vi "Actuator.vi"(10 "Actuator":bool, 11 "lines":tag) -> ()   [LabVIEW 2016]
uses:
  <vilib>/DAQmx/write.llb/DAQmx Write (Digital Bool 1Line 1Point).vi
  <vilib>/DAQmx/create/channels.llb/DAQmx Create Channel (DO-Digital Output).vi
  <vilib>/DAQmx/miscellaneous.llb/DAQmx Fill In Error Info.vi
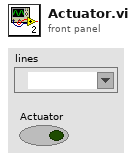
[diagram p1: front panel]
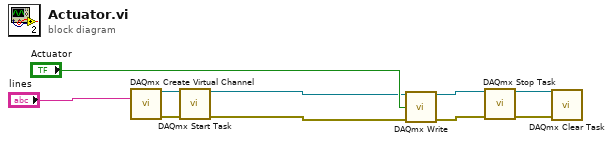
[diagram p0: block diagram]
diagram:
  n1 = call-poly <vilib>:"DAQmx Create Virtual Channel.vi"("lines"="lines") -> ("task out"=w2:refnum<k21>, "error out"=w6:errorcluster)  [unwired: 13 in]
  n2 = call <vilib>:"DAQmx Start Task.vi"("task/channels in"=w2, "error in"=w6) -> ("task out"=w3:refnum<k21>, "error out"=w7:errorcluster)  [unwired: 12 in]
  n3 = call-poly <vilib>:"DAQmx Write.vi"("task/channels in"=w3, "data"="Actuator", "error in"=w7) -> ("task out"=w4:refnum<k21>, "error out"=w8:errorcluster)  [unwired: 10 in, 1 out]
  n4 = call <vilib>:"DAQmx Stop Task.vi"("task/channels in"=w4, "error in"=w8) -> ("task out"=w5:refnum<k21>, "error out"=w9:errorcluster)  [unwired: 12 in]
  n5 = call <vilib>:"DAQmx Clear Task.vi"("task in"=w5, "error in"=w9) -> ()  [unwired: 13 in, 1 out]
